vi "to_json.vi"(8 "error in":errorcluster, 11 "include in":refnum<class "include.lvclass">) -> (0 "error out":errorcluster, 2 "json":string, 3 "include out":refnum<class "include.lvclass">)   [LabVIEW 2020, in "nominal types.lvlib" / "channelFilter.lvlib" / "include.lvclass"]
uses:
  include.lvclass
  include.lvclass/include.ctl
  <vilib>/JDP Science/JSONtext/support/Format JSON Array Text.vi
  <vilib>/JDP Science/JSONtext/support/Format JSON Object.vi
  <vilib>/JDP Science/JSONtext/JSONtext.lvlib
  b423daf5-c2a3-4c24-a941-a75b541187cf.vi
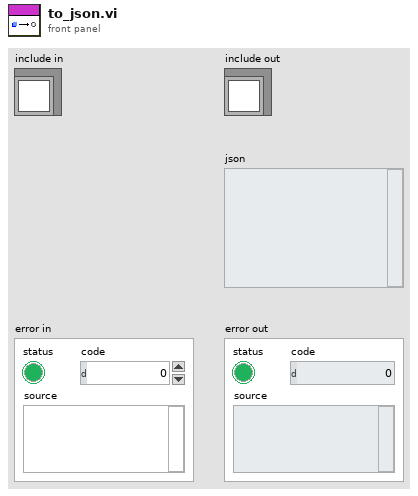
[diagram p1: front panel]
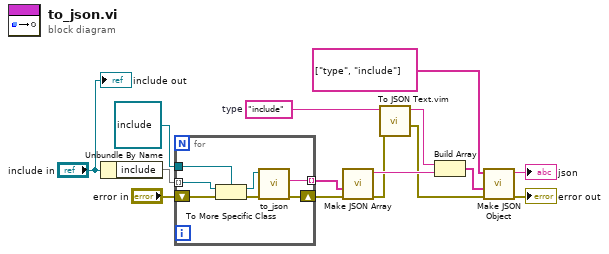
[diagram p0: block diagram]
diagram:
  w8 = "include"  # type
  n1 = Unbundle By Name("include in") -> ("include"=w14:set{refnum<class>})
  n2 = for {
    tunnel: w14 -> [w22] mode=indexing
    tunnel: refnum<class "include.lvclass"> refnum ("nominal types.lvlib:channelFilter.lvlib:include.lvclass") -> [w21]
    tunnel: [w19] -> w11 mode=indexing
    shift-right: [w17] -> w10
    shift-left: "error in" -> [w16]
    n3 = To More Specific Class(target class=w21, reference=w22, error in=w16) -> (specific class reference=w20:refnum<class "include.lvclass">, error out=w18:errorcluster)
    n4 = call-dynamic "to_json.vi"("error in"=w18, "include in"=w20) -> ("error out"=w17:errorcluster, "json"=w19:string)  [unwired: 7 in, 1 out]
  }
  n5 = call <vilib>:"Make JSON Array.vi"("error in (no error)"=w10, "JSON Elements"=w11) -> ("error out"=w2:errorcluster, "<JSON>"=w7:string)  [unwired: 8 in]
  n6 = call "To JSON Text.vim"("error in (no error)"=w2, "Anything"=w8) -> ("error out"=w1:errorcluster, "<JSON>"=w3:string)  [unwired: 8 in]
  n7 = Build Array(w3, w7) -> (w6:string[])
  n8 = call <vilib>:"Make JSON Object.vi"("error in (no error)"=w1, "JSON Items"=w6, "Item Names"=string[] ["type", "include"]) -> ("error out"=→"error out":errorcluster, "<JSON>"=→"json":string)  [unwired: 7 in]
  "include out" <- "include in"
